vi "Apply Config.vi"(8 "error in":errorcluster, 10 "Data":T1 {"Outport Channel refs" format="%.0x"; "Inport Channel refs" format="%.0x"}, 11 "Compiled.Settings in":T1 {"Outport Channel refs" format="%.0x"; "Inport Channel refs" format="%.0x"}) -> (0 "error out":errorcluster, 3 "Compiled.Settings out":T1 {"Outport Channel refs" format="%.0x"; "Inport Channel refs" format="%.0x"})   [LabVIEW 2025, in "Runtime Configuration Support Example Engine.lvlib"]
uses:
  Runtime Configuration Support Example Engine.lvlib
  Shared/Compiled.Settings.ctl
  <vilib>/NI VeriStand/Custom Device API/Custom Device Item Ref.ctl
  <vilib>/NI VeriStand/Custom Device API/Custom Device API.lvlib
  Shared/Runtime Configuration Support Example Shared.lvlib
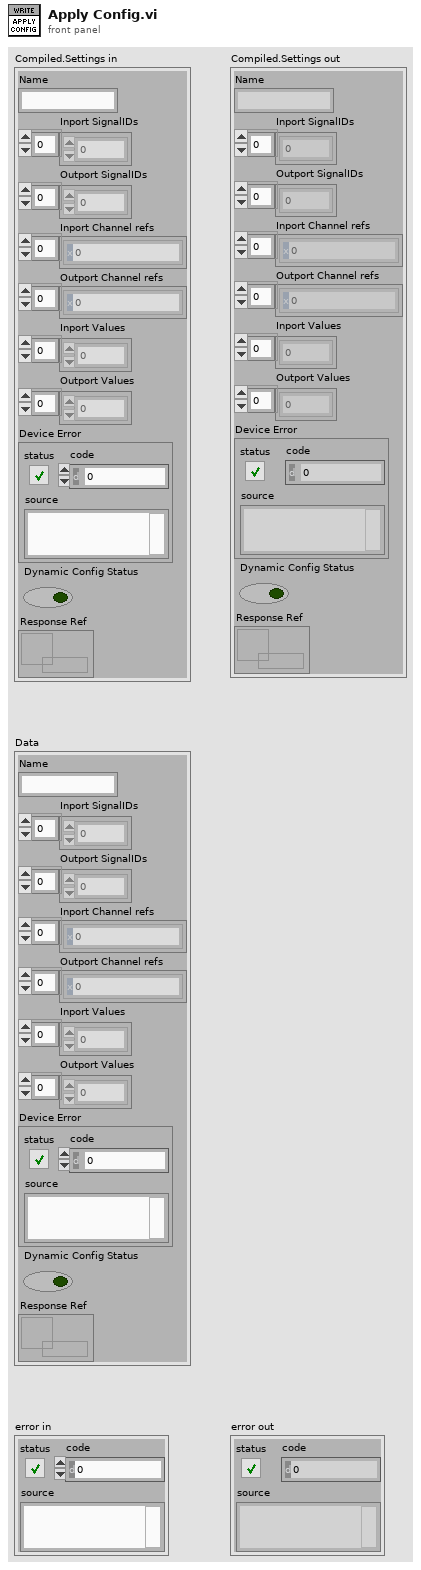
[diagram p1: front panel]
types:
  T1 = typedef "Runtime Configuration Support Example Shared.lvlib/Compiled.Settings.ctl" = cluster{"Name":string, "Inport SignalIDs":i32[], "Outport SignalIDs":i32[], "Inport Channel refs":T2[], "Outport Channel refs":T2[], "Inport Values":dbl[], "Outport Values":dbl[], "Device Error":errorcluster, "Dynamic Config Status":bool, "Response Ref":refnum<queue>}
  T2 = typedef "Custom Device API.lvlib/Custom Device Item Ref.ctl" = u64
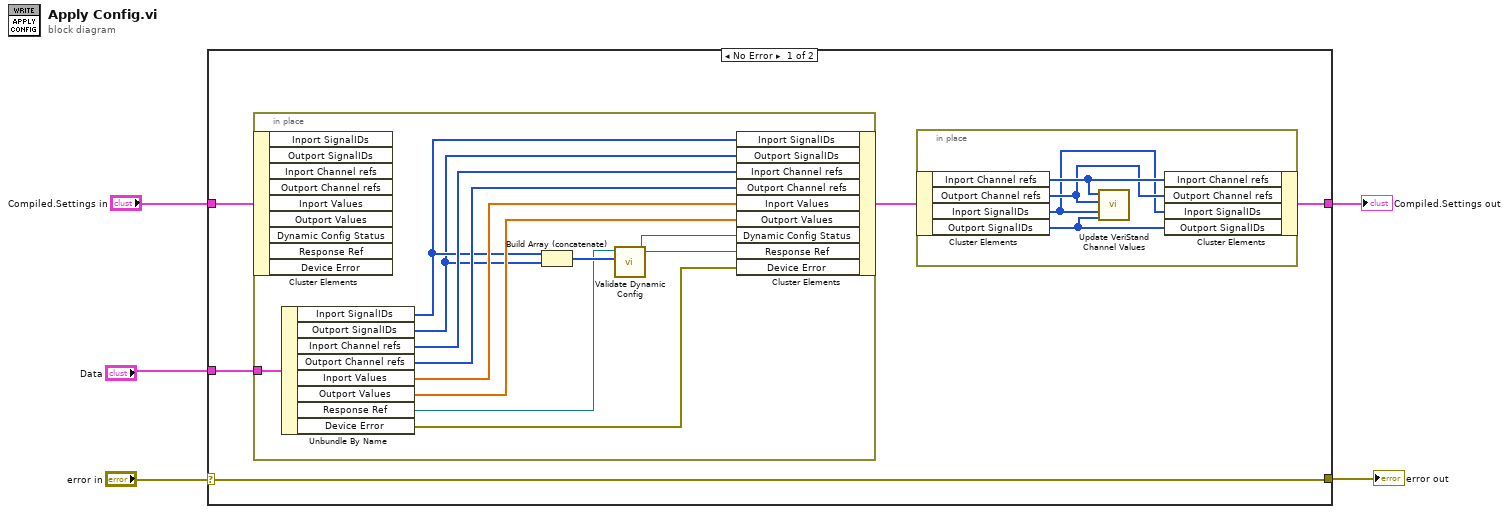
[diagram p0: block diagram]
diagram:
  n1 = case shown="No Error" "error in" {
    selector: "error in" -> [w10 w28]
    tunnel: [w6 w27] -> w3
    tunnel: "Compiled.Settings in" -> [w9 w27]
    tunnel: "Data" -> [w8 _]
    tunnel: [w10 w28] -> w5
    frame No Error {
      n2 = in-place {
        in-place-border: w8 -> [w23]
        n3 = in-place-cluster #1(w9) -> ()  [unwired: 9 out]
        n4 = Unbundle By Name(w23) -> ("Inport SignalIDs"=w19:i32[], "Outport SignalIDs"=w18:i32[], "Inport Channel refs"=w25:T2[], "Outport Channel refs"=w24:T2[], "Inport Values"=w21:dbl[], "Outport Values"=w20:dbl[], "Response Ref"=w17:refnum<queue>, "Device Error"=w26:errorcluster)
        n5 = Build Array (concatenate)(w19, w18) -> (w22:i32[])
        n6 = call "Validate Dynamic Config.vi"("SignalIDs"=w22, "Response Ref in"=w17) -> ("Response Ref  out"=w15:refnum<queue>, "Dynamic Config Status"=w16:bool)  [unwired: 8 in]
        n7 = in-place-cluster #1("Inport SignalIDs"=w19, "Outport SignalIDs"=w18, "Inport Channel refs"=w25, "Outport Channel refs"=w24, "Inport Values"=w21, "Outport Values"=w20, "Dynamic Config Status"=w16, "Response Ref"=w15, "Device Error"=w26) -> (w7:T1)
      }
      n8 = in-place {
        n9 = in-place-cluster #2(w7) -> ("Inport Channel refs"=w14:T2[], "Outport Channel refs"=w12:T2[], "Inport SignalIDs"=w11:i32[], "Outport SignalIDs"=w13:i32[])
        n10 = call "Update VeriStand Channel Values.vi"("SignalIds Out"=w13, "SignalIds In"=w11, "Outport Channel refs"=w12, "Inport Channel refs"=w14) -> ()  [unwired: 8 in]
        n11 = in-place-cluster #2("Inport Channel refs"=w14, "Outport Channel refs"=w12, "Inport SignalIDs"=w11, "Outport SignalIDs"=w13) -> (w6:T1)
      }
    }
    frame Error {
    }
  }
  "Compiled.Settings out" <- w3
  "error out" <- w5
